vi "convert_stringArray_to_string.vi"(2 "Max Elements Count (All)":i32=-1, 4 "string array in":string[](array[string]), 5 "String to add before (\"\")":string) -> (1 "string out":string)   [LabVIEW 2014, in "rszvl_rsidr_core.lvlib"]
uses:
  rszvl_rsidr_core.lvlib
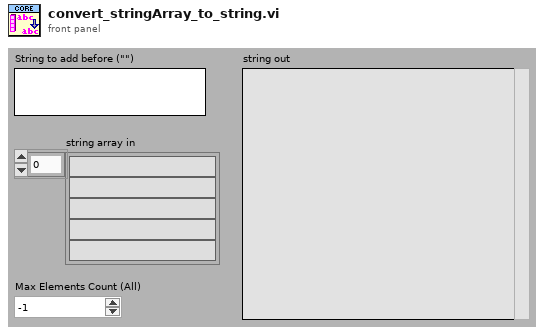
[diagram p1: front panel]
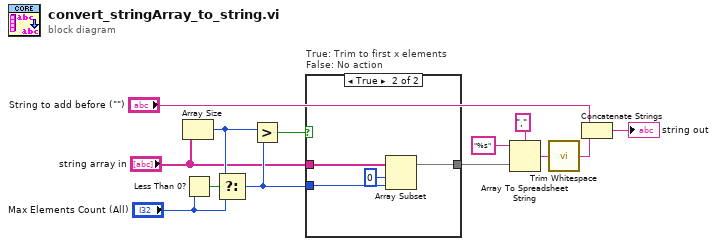
[diagram p0: block diagram]
diagram:
  n1 = Array Size(array="string array in") -> (size(s)=w3:i32)
  n2 = Less Than 0?(x="Max Elements Count (All)") -> (x < 0?=w7:bool)
  n3 = Select(t=w3, s=w7, f="Max Elements Count (All)") -> (s? t:f=w4:i32)
  n4 = Greater?(x=w3, y=w4) -> (0:w5:bool)
  n5 = case "True: Trim to first x elements\nFalse: No action" shown="True" w5 {
    tunnel: [w14 w15] -> w1
    tunnel: "string array in" -> [w14 w18]
    tunnel: w4 -> [_ w16]
    frame False {
    }
    frame True {
      n6 = Array Subset(array=w18, index=0, length=w16) -> (w15:string[])
    }
  }
  n7 = Array To Spreadsheet String(delimiter (Tab)=",", array=w1, 3:"%s" ("format string")) -> (spreadsheet string=w11:string)
  n8 = call "Trim Whitespace.vi"("string"=w11) -> ("trimmed string"=w9:string)  [unwired: 1 in]
  n9 = Concatenate Strings("String to add before (\"\")", w9) -> (→"string out":string)
